vi "2.vi"() -> ()   [LabVIEW 2017]
uses:
  <vilib>/Instr/_visa.llb/VISA Configure Serial Port (Instr).vi
panel:
  in  "停止":bool
  out "波形图表":i32(graph)
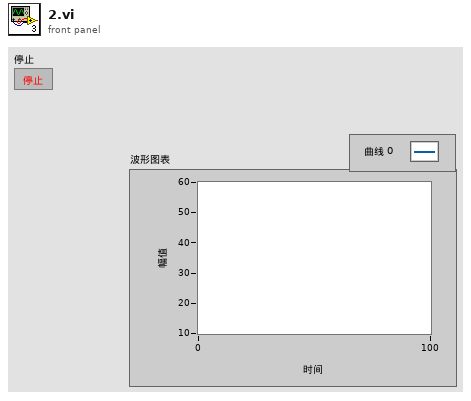
[diagram p1: front panel]
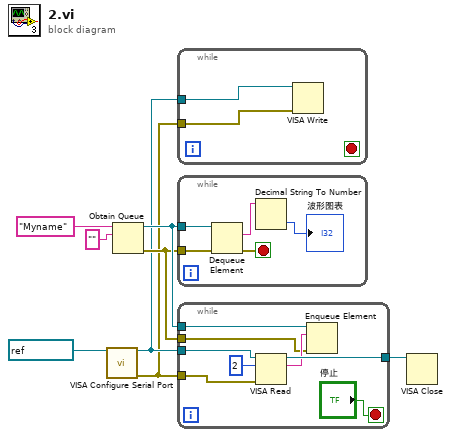
[diagram p0: block diagram]
diagram:
  n1 = call-poly "VISA Configure Serial Port"("VISA resource name"=refnum<visa-resource-name> "COM2") -> ("VISA resource name out"=w2:refnum<visa-resource-name>, "error out"=w1:errorcluster)  [unwired: 13 in]
  n2 = Obtain Queue(name (unnamed)="Myname" ("名称（未命名）"), element data type="") -> (queue out=w5:refnum<queue>, error out=w3:errorcluster)  [unwired: 3 in, 1 out]
  n3 = while {
    tunnel: w2 -> [w10]
    tunnel: w1 -> [w9]
    stop <- _ stop-if-true
    n4 = VISA Write(VISA resource name=w10, error in (no error)=w9) -> ()  [unwired: 1 in, 3 out]
  }
  n5 = while {
    tunnel: w5 -> [w15]
    tunnel: w3 -> [w12]
    stop <- w11 stop-if-true
    n6 = Dequeue Element(queue=w15, error in (no error)=w12) -> (element=w14:string, error out=w11:errorcluster)  [unwired: 1 in, 2 out]
    n7 = Decimal String To Number(string=w14) -> (number=→"波形图表":i32)  [unwired: 2 in, 1 out]
  }
  n8 = while {
    tunnel: w2 -> [w23]
    tunnel: [w22] -> w8
    tunnel: w5 -> [w19]
    tunnel: w3 -> [w17]
    tunnel: w1 -> [w16]
    stop <- "停止" stop-if-true
    n9 = VISA Read(VISA resource name=w23, byte count=u32 2 ("字节总数"), error in (no error)=w16) -> (VISA resource name out=w22:refnum<visa-resource-name>, read buffer=w20:string)  [unwired: 2 out]
    n10 = Enqueue Element(queue=w19, element=w20, error in (no error)=w17) -> ()  [unwired: 1 in, 3 out]
  }
  n11 = VISA Close(VISA resource name=w8) -> ()  [unwired: 1 in, 1 out]
